vi "GT Get Sts.vi"(6 "pClock":u32, 7 "count":i16, 8 "error in (no error)":errorcluster caption="错误输入（无错误）", 10 "axis":i16, 11 "cardNum":i16) -> (0 "error out":errorcluster caption="错误输出", 2 "pSts 2":i32, 3 "function return":i16, 4 "pClock out":u32)   [LabVIEW 2020, in "gts.lvlib"]
doc: "GT_API GT_GetSts(short cardNum,short axis,long *pSts,short count=1,unsigned long *pClock=NULL);"
uses:
  gts.lvlib
  dll/32bit/multi_card/gts.dll
panel:
  in  "pSts":i32
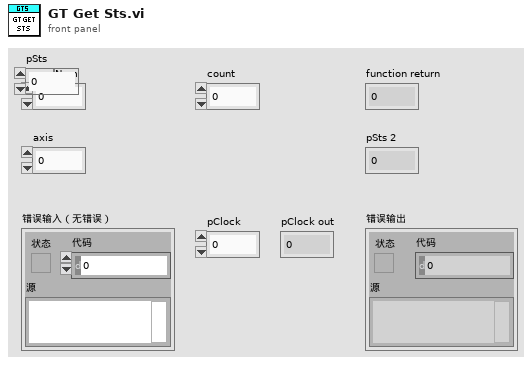
[diagram p1: front panel]
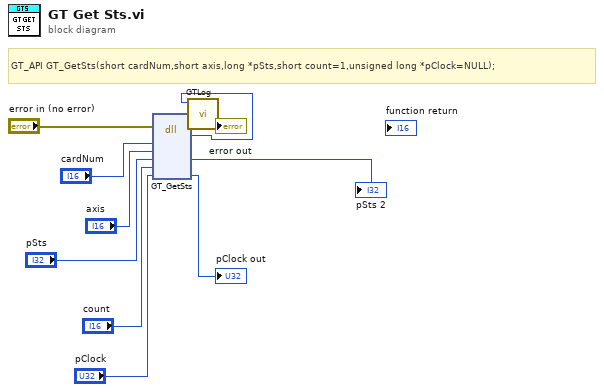
[diagram p0: block diagram]
diagram:
  # "GT_API GT_GetSts(short cardNum,short axis,long *pSts,short count=1,unsigned long *pClock=NULL);"
  n1 = dll-call lib="C:/1228/dll/32bit/multi_card/gts.dll" fn="GT_GetSts"(error in="error in (no error)", "cardNum"="cardNum", "axis"="axis", "pSts"="pSts", "count"="count", "pClock"="pClock") -> (error out=w5:errorcluster, "返回类型"=w1:i16, "pSts"=→"pSts 2":i32, "pClock"=→"pClock out":u32)  [unwired: 5 in, 1 out]
  n2 = call "GTLog.vi"("error in (no error)"=w5, "Numeric"=w1) -> ("error out"=→"error out":errorcluster)  [unwired: 9 in]
